vi "A2L Get DAQ List ID.vi"(8 "error in (no error)":errorcluster, 11 "ECU ref in":T1) -> (0 "error out":errorcluster, 2 "DAQ List IDs":u32[](array[numeric]) format="%.0x", 3 "ECU ref out":T1)   [LabVIEW 2019, in "A2L Utility.lvlib"]
uses:
  A2L Utility.lvlib
  <vilib>/ECUMC/ECUMC.llb/MC Reference.ctt
  Private/ParseNumeric.vi
  <vilib>/ECUMC/ECUMC.llb/MC Get Prop DB File Name.vi
  <vilib>/Utility/file.llb/Read Delimited Spreadsheet (string).vi
  <vilib>/Utility/error.llb/Error Cluster From Error Code.vi
  <vilib>/ECUMC/ECUMC.lvlib
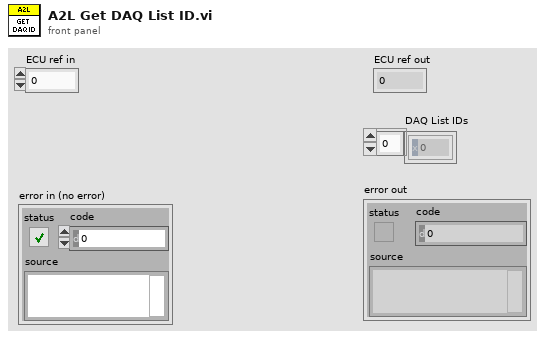
[diagram p1: front panel]
types:
  T1 = typedef "ECUMC.lvlib/MC Reference.ctt" = u32
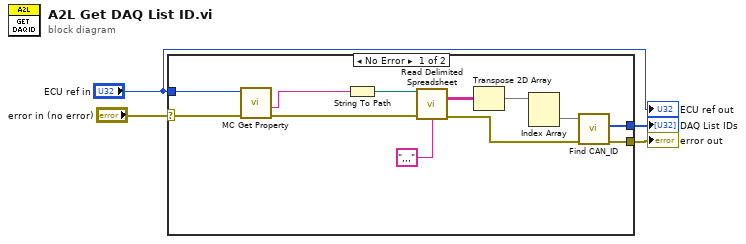
[diagram p0: block diagram]
diagram:
  n1 = case shown="No Error" "error in (no error)" {
    selector: "error in (no error)" -> [w10 w17]
    tunnel: "ECU ref in" -> [w11 _]
    tunnel: [w7 w17] -> w3
    tunnel: [w5 _] -> w1
    frame No Error {
      n2 = call-poly <vilib>:"MC Get Property.vi"("error in"=w10, "reference in"=w11) -> ("error out"=w12:errorcluster, "DB file name"=w6:string)  [unwired: 7 in, 1 out]
      n3 = String To Path(string=w6) -> (path=w16:path)
      n4 = call-poly <vilib>:"Read Delimited Spreadsheet.vi"("file path (dialog if empty)"=w16, "error in (no error)"=w12, "delimiter (\\t)"=",,," ("delimiter (\\t)")) -> ("all rows"=w14:string[][], "error out"=w9:errorcluster)  [unwired: 7 in, 4 out]
      n5 = Transpose 2D Array(2D array=w14) -> (transposed array=w13:string[][])
      n6 = Index Array(array=w13) -> (element=w8:string[])  [unwired: 2 in]
      n7 = call "Find CAN_ID.vi"("error in (no error)"=w9, "A2L Text In"=w8) -> ("error out"=w7:errorcluster, "DTO_ID"=w5:u32[])  [unwired: 8 in]
    }
    frame Error {
    }
  }
  "error out" <- w3
  "DAQ List IDs" <- w1
  "ECU ref out" <- "ECU ref in"
